vi "History Retrieve Record.vi"(8 "error in (no error)":errorcluster, 11 "Statement Refnum":T1) -> (0 "error out":errorcluster, 2 "History Record":T2, 3 "Statement Refnum":T1)   [LabVIEW 2011]
uses:
  History Record.ctl
  Summitek EXT/ODBC/SQL Controls/Statement Refnum.ctl
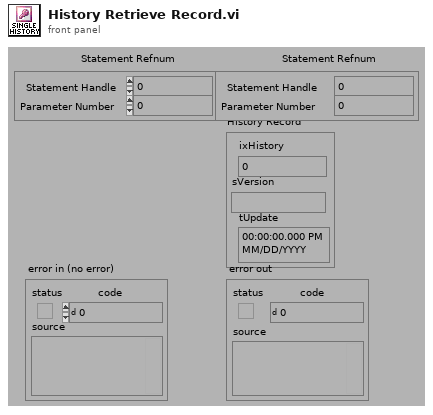
[diagram p1: front panel]
types:
  T1 = typedef "Statement Refnum.ctl" = cluster{"Statement Handle":i32, "Parameter Number":u16}
  T2 = typedef "History Record.ctl" = cluster{"ixHistory":i32, "sVersion":string, "tUpdate":timestamp}
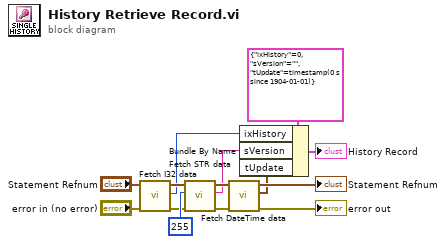
[diagram p0: block diagram]
diagram:
  n1 = call "Fetch I32 data.vi"("error in (no error)"="error in (no error)", "Statement Refnum"="Statement Refnum") -> ("error out"=w8:errorcluster, "Data"=w3:i32, "Statement Refnum"=w9:T1)  [unwired: 3 out]
  n2 = call "Fetch STR data.vi"("error in (no error)"=w8, "Buffer Size"=255, "Statement Refnum"=w9) -> ("error out"=w6:errorcluster, "Data"=w2:string, "Statement Refnum"=w7:T1)  [unwired: 2 out]
  n3 = call "Fetch DateTime data.vi"("error in (no error)"=w6, "Statement Refnum"=w7) -> ("error out"=→"error out":errorcluster, "Data"=w1:timestamp, "Statement Refnum"=→"Statement Refnum":T1)  [unwired: 3 out]
  n4 = Bundle By Name(cluster=T2 {"ixHistory"=0, "sVersion"="", "tUpdate"=timestamp(0 s since 1904-01-01)} ("Field Data Information"), "ixHistory"=w3, "sVersion"=w2, "tUpdate"=w1) -> (→"History Record":T2)
